vi "ConsoleApplication.vi"(5 "Source Directory":path, 6 "error in":errorcluster, 7 "filename":string="__main__.py", 8 "parser name":string="parser", 9 "VI Interpreter":refnum<class "VI Interpreter.lvclass">) -> (0 "error out":errorcluster, 3 "VI Interpreter out":refnum<class "VI Interpreter.lvclass">, 4 "python":string)   [LabVIEW 2014, in "PyConvBD.lvclass"]
uses:
  PyConvBD.lvclass
  VI Interpreter/Classes/VI Interpreter/VI Interpreter.lvclass
  Parsing/Python Functions.lvlib
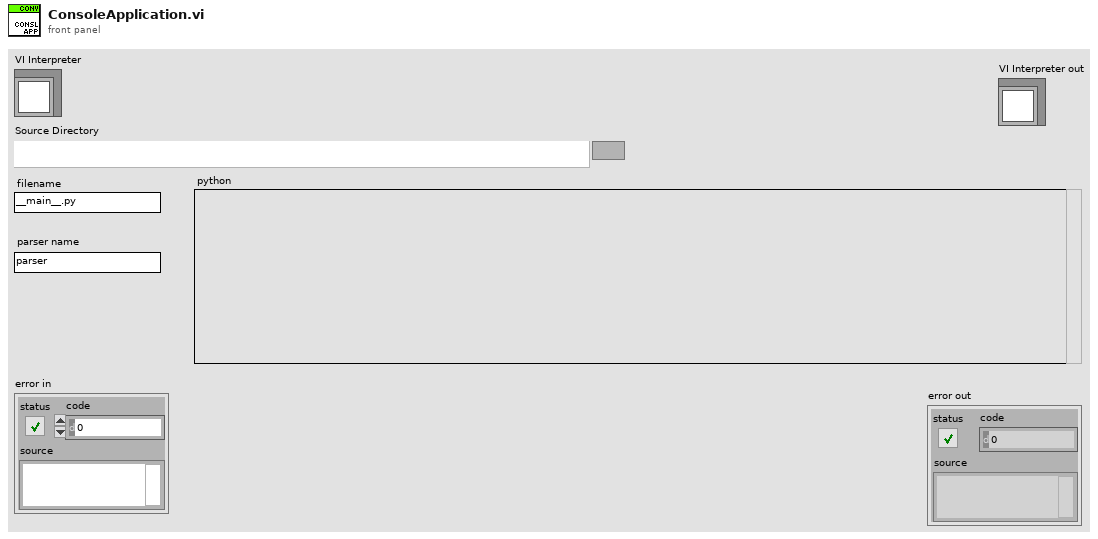
[diagram p1: front panel]
types:
  T1 = typedef "ConsoleArg_TD.ctl" = cluster{"position":i32, "order":i32, "flags":string[], "description":string, "required":bool, "type":variant, "label":string}
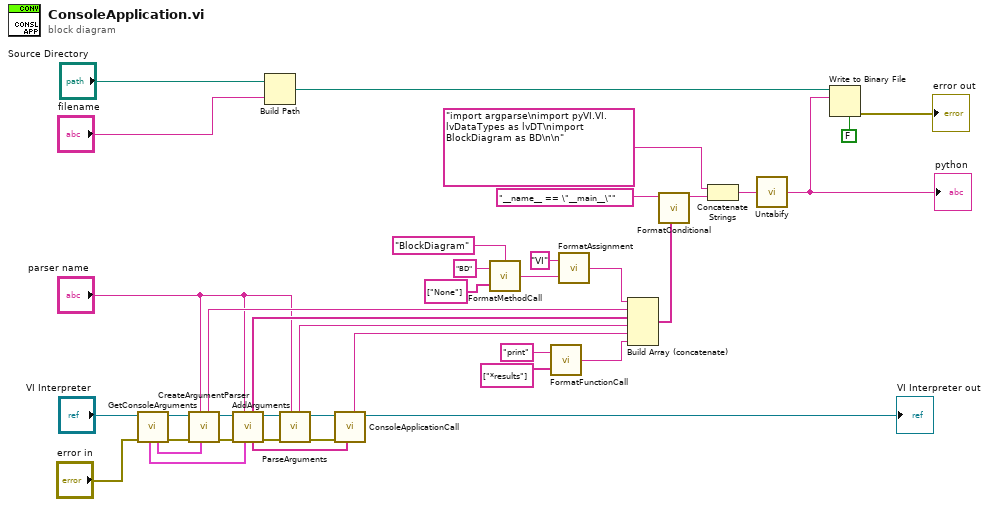
[diagram p0: block diagram]
diagram:
  n1 = call "GetConsoleArguments.vi"("error in"="error in", "VI Interpreter"="VI Interpreter") -> ("error out"=w29:errorcluster, "VI Interpreter out"=w31:refnum<class "VI Interpreter.lvclass">, "outputs"=w30:T1[], "inputs"=w26:T1[])  [unwired: 4 in]
  n2 = call "CreateArgumentParser.vi"("outputs"=w30, "parser name"="parser name", "error in"=w29, "VI Interpreter in"=w31) -> ("error out"=w27:errorcluster, "VI Interpreter out"=w28:refnum<class "VI Interpreter.lvclass">, "python assignment"=w35:string)  [unwired: 5 in]
  n3 = call "AddArguments.vi"("inputs"=w26, "parser name"="parser name", "error in"=w27, "VI Interpreter in"=w28) -> ("error out"=w23:errorcluster, "VI Interpreter out"=w24:refnum<class "VI Interpreter.lvclass">, "names"=w9:string[], "arguments"=w25:string[])  [unwired: 4 in]
  n4 = Build Path(base path="Source Directory", name or relative path="filename") -> (appended path=w13:path)
  n5 = call "ParseArguments.vi"("parser name"="parser name", "error in"=w23, "VI Interpreter in"=w24) -> ("error out"=w10:errorcluster, "VI Interpreter out"=w11:refnum<class "VI Interpreter.lvclass">, "python assignment"=w21:string)  [unwired: 6 in]
  n6 = call "ConsoleApplicationCall.vi"("names"=w9, "error in"=w10, "VI Interpreter in"=w11) -> ("VI Interpreter out"=→"VI Interpreter out":refnum<class "VI Interpreter.lvclass">, "Call"=w8:string)  [unwired: 6 in, 1 out]
  n7 = call "FormatMethodCall.vi"("method"="BlockDiagram" ("object"), "parameters"=string[] ["None"], "object"="BD" ("method")) -> ("python object"=w15:string)
  n8 = call "FormatFunctionCall.vi"("parameters"=string[] ["*results"], "function"="print") -> ("python object"=w5:string)
  n9 = call "FormatAssignment.vi"("value"=w15, "name"="VI") -> ("python assignment"=w17:string)
  n10 = Build Array (concatenate)(w17, w35, w25, w21, w8, w5) -> (w34:string[])
  n11 = call "FormatConditional.vi"("if"=w34, "condition"="__name__ == \"__main__\"") -> ("python"=w20:string)  [unwired: 7 in]
  n12 = Concatenate Strings("import argparse\nimport pyVI.VI.lvDataTypes as lvDT\nimport BlockDiagram as BD\n\n" ("string"), w20) -> (w19:string)
  n13 = call "Untabify.vi"("string in"=w19) -> ("string out"=w12:string)  [unwired: 1 in]
  "python" <- w12
  n14 = Write to Binary File(file (use dialog)=w13, data=w12, 5:FALSE ("prepend array or string size? (T)")) -> (error out=→"error out":errorcluster)  [unwired: 3 in, 2 out]
